vi "Error Output.vi"() -> ()   [LabVIEW 2010]
doc: "This VI is used to demonstrate undefined data."
panel:
  out "Waveform Graph":dynamicdata(graph) caption="Sine"
  in  "Frequency":dbl=nan
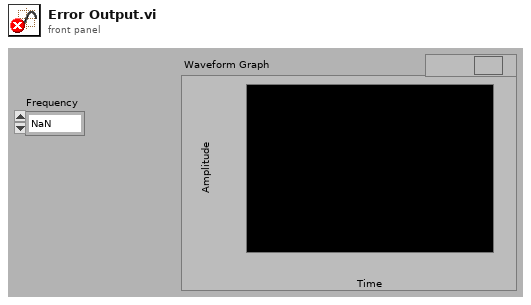
[diagram p1: front panel]
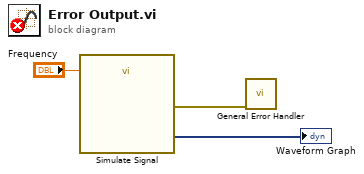
[diagram p0: block diagram]
diagram:
  n1 = call "Simulate Signal"("Frequency"="Frequency") -> ("Sine"=→"Waveform Graph":dynamicdata, "error out"=w1:errorcluster)  [unwired: 13 in]
  n2 = call <vilib>:"General Error Handler.vi"("error in (no error)"=w1) -> ()  [unwired: 10 in, 5 out]
